vi "controller.vi"(8 "error in (no error)":errorcluster, 9 "y":dbl, 10 "Setpoint":dbl, 11 "Cluster":T1={"Transfer Function"={"Numerator"=[1.0], "Denominator"=[-0.9, 1.0]}, "Limit Cluster"={"Upper Limit"=0.0, "Lower Limit"=0.0}}) -> (0 "error out":errorcluster, 2 "Uncoerced Output":dbl, 3 "Output":dbl)   [LabVIEW 2020]
uses:
  Controls/controlspec.ctl
  <vilib>/Simulation/DiscreteLinear/Implementation/NILVSim Discrete Transfer Function Direct.llb/SIM Discrete Transfer Function Diagram (SISO).vi
  <vilib>/Simulation/ContinuousLinear/Implementation/Shared/SIM Transfer Function Support.llb/SIM TransferFunction Normalize to Buffer.vi
  <vilib>/Simulation/DiscreteLinear/Implementation/Shared/SIM Init Discrete States.vi
  <vilib>/Simulation/DiscreteLinear/Implementation/NILVSim Discrete Transfer Function Direct.llb/SIM Transfer Function Direct core (SISO).vi
  <vilib>/Simulation/ContinuousLinear/Implementation/Shared/SIM Transfer Function Support.llb/SIM TransferFunction Normalize.vi
  <vilib>/Simulation/Implementation/Shared/SIM Polynomials.llb/SIM Remove Zero Coefficients (DBL).vi
  <vilib>/Simulation/Implementation/Shared/SIM Polynomials.llb/SIM Divide Polynomials (DBL).vi
  <vilib>/Simulation/Implementation/Shared/SIM BuildSimErr.vi
  <vilib>/Simulation/Implementation/XNodeFramework/SimXNode/SimX.xnode
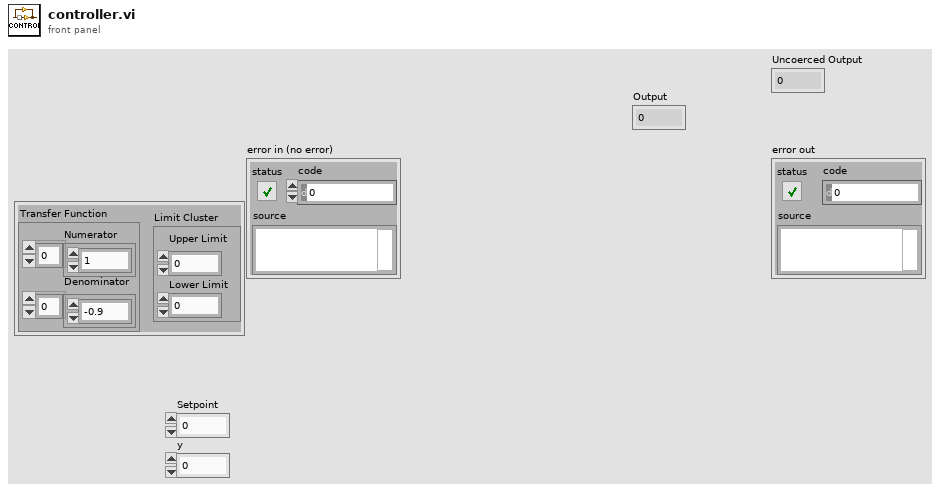
[diagram p1: front panel]
types:
  T1 = typedef "controlspec.ctl" = cluster{"Transfer Function":cluster{"Numerator":dbl[], "Denominator":dbl[]}, "Limit Cluster":cluster{"Upper Limit":dbl, "Lower Limit":dbl}}
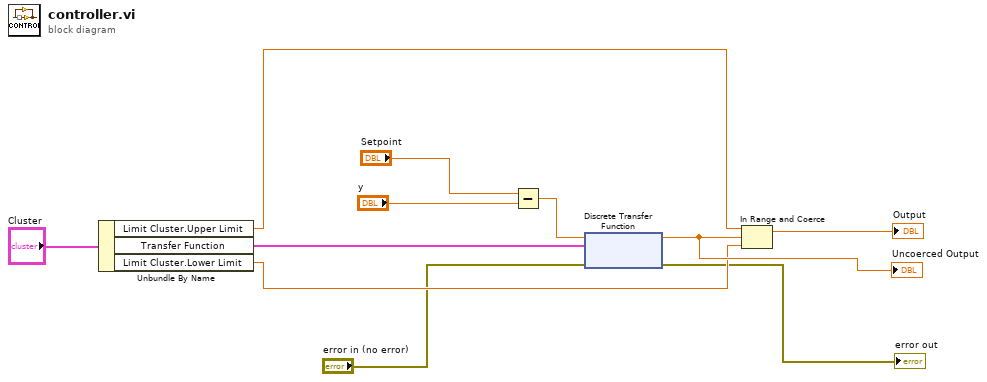
[diagram p0: block diagram]
diagram:
  n1 = Unbundle By Name("Cluster") -> ("Limit Cluster.Upper Limit"=w5:dbl, "Transfer Function"=w4:cluster{"Numerator":dbl[], "Denominator":dbl[]}, "Limit Cluster.Lower Limit"=w3:dbl)
  n2 = Subtract(x="Setpoint", y="y") -> (x-y=w10:dbl)
  n3 = xnode ("Discrete Transfer Function")("input u(k)"=w10, "Transfer Function"=w4, "error in (no error)"="error in (no error)") -> ("output y(k)"=w11:dbl, "error out"=→"error out":errorcluster)  [unwired: 1 in]
  "Uncoerced Output" <- w11
  n4 = In Range and Coerce(upper limit=w5, x=w11, lower limit=w3) -> (coerced(x)=→"Output":dbl)  [unwired: 1 out]
